vi "Tank Fill.vi"() -> ()   [LabVIEW 2014]
panel:
  out "Tank Level N":i32
  in  "Stop Fill":bool
  in  "Start Fill":bool
  out "Bottom Float Switch":bool
  out "Top Float Switch":bool
  out "Tank level":i32(slide) scale=0.0..300.0
  # "Click          to run"
  # "225"
  # "75"
  # "Tank Fill"
  # "Here, there is a 300 gallon mix tank which mixes red dye.  It drains at a constant rate of 50 gal/sec. There is a pump that can add dye at a rate of 100 gal/sec.\nThere are two float switches, which monitor the level in the tank. When the dye level reaches one of the switches, it is activated, and its value becomes true.\n\nYour job is to add this functionality:\nThe pump is activated by the Start Fill button. When this starts, dye gets pumped into the mix tank until it hits the top float switch. Once this switch is reached, the pump turns off.  \nThe tank level decreases until it the level goes below the bottom float switch. At this point, the pump should start back up and restart the cycle. The tank level should oscillate between the two float switches like this until the stop fill button is pushed, at which point the tank will drain."
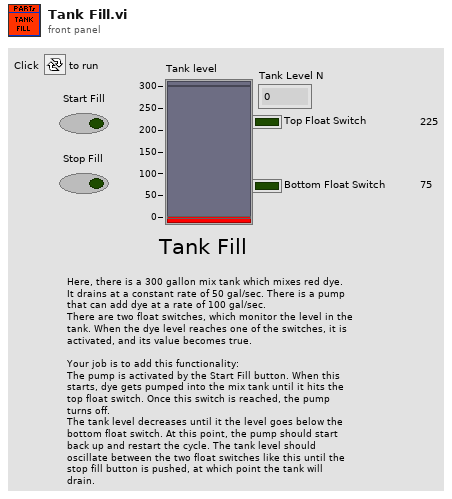
[diagram p1: front panel]
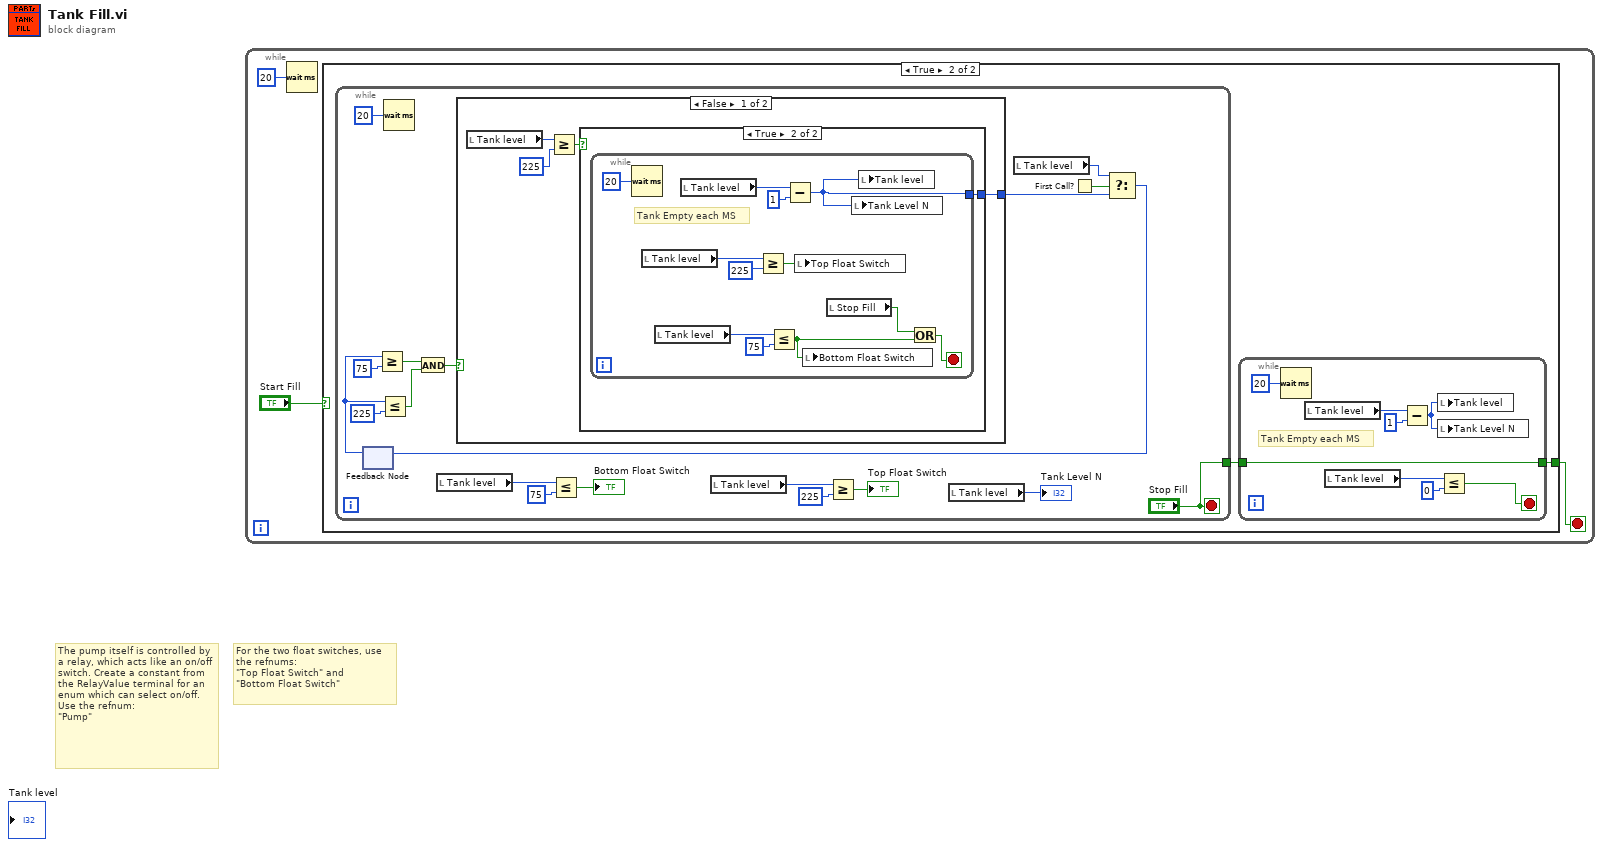
[diagram p0: block diagram]
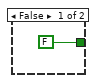
[diagram p2: hidden frame]
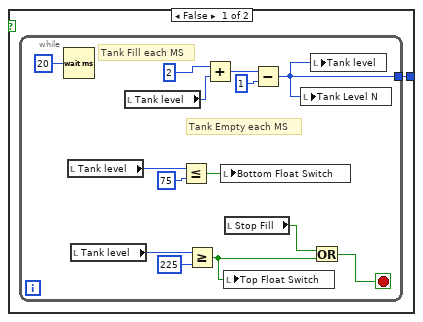
[diagram p3: hidden frame]
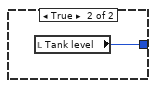
[diagram p4: hidden frame]
diagram:
  # "The pump itself is controlled by a relay, which acts like an on/off switch. Create a constant from the RelayValue terminal for an enum which can select on/off.\nUse the refnum:\n\"Pump\""
  # "For the two float switches, use\nthe refnums:\n\"Top Float Switch\" and\n\"Bottom Float Switch\""
  n1 = while {
    stop <- w2 stop-if-true
    n2 = Wait (ms)(milliseconds to wait=u32 20) -> ()  [unwired: 1 out]
    n3 = case shown="True" "Start Fill" {
      tunnel: [FALSE ("Stop Fill") w5] -> w2
      frame False {
      }
      frame True {
        n4 = while {
          tunnel: ["Stop Fill"] -> w6
          stop <- "Stop Fill" stop-if-true
          n5 = feedback #1() -> (w18:i32)  [unwired: 1 in]
          n6 = Greater Or Equal?(x=w18, y=75) -> (x >= y?=w25:bool)
          n7 = Less Or Equal?(x=w18, y=225) -> (x <= y?=w24:bool)
          n8 = Wait (ms)(milliseconds to wait=u32 20) -> ()  [unwired: 1 out]
          n9 = And(x=w25, y=w24) -> (x .and. y?=w23:bool)
          n10 = local read "Tank level"() -> (w30:i32)
          n11 = case shown="False" w23 {
            tunnel: [w34 w66] -> w20
            frame False {
              n12 = local read "Tank level"() -> (w37:i32)
              n13 = Greater Or Equal?(x=w37, y=225) -> (x >= y?=w35:bool)
              n14 = case shown="True" w35 {
                tunnel: [w38 w53] -> w34
                frame False {
                  n15 = while {
                    tunnel: [w40] -> w38
                    stop <- w41 stop-if-true
                    # "Tank Empty each MS"
                    # "Tank Fill each MS"
                    n16 = Wait (ms)(milliseconds to wait=u32 20) -> ()  [unwired: 1 out]
                    n17 = local read "Tank level"() -> (w45:i32)
                    n18 = local read "Tank level"() -> (w52:i32)
                    n19 = local read "Tank level"() -> (w50:i32)
                    n20 = Less Or Equal?(x=w45, y=75) -> (x <= y?=w44:bool)
                    n21 = Greater Or Equal?(x=w52, y=225) -> (x >= y?=w42:bool)
                    n22 = Add(x=2, y=w50) -> (x+y=w49:i32)
                    n23 = local write "Bottom Float Switch"(w44) -> ()
                    n24 = local write "Top Float Switch"(w42) -> ()
                    n25 = local read "Stop Fill"() -> (w43:bool)
                    n26 = Subtract(x=w49, y=1) -> (x-y=w40:i32)
                    n27 = local write "Tank Level N"(w40) -> ()
                    n28 = local write "Tank level"(w40) -> ()
                    n29 = Or(x=w43, y=w42) -> (x .or. y?=w41:bool)
                  }
                }
                frame True {
                  n30 = while {
                    tunnel: [w58] -> w53
                    stop <- w60 stop-if-true
                    # "Tank Empty each MS"
                    n31 = Wait (ms)(milliseconds to wait=u32 20) -> ()  [unwired: 1 out]
                    n32 = local read "Tank level"() -> (w56:i32)
                    n33 = local read "Tank level"() -> (w65:i32)
                    n34 = local read "Tank level"() -> (w61:i32)
                    n35 = Greater Or Equal?(x=w56, y=225) -> (x >= y?=w54:bool)
                    n36 = Less Or Equal?(x=w65, y=75) -> (x <= y?=w57:bool)
                    n37 = Subtract(x=w61, y=1) -> (x-y=w58:i32)
                    n38 = local write "Top Float Switch"(w54) -> ()
                    n39 = local write "Bottom Float Switch"(w57) -> ()
                    n40 = local read "Stop Fill"() -> (w59:bool)
                    n41 = local write "Tank Level N"(w58) -> ()
                    n42 = local write "Tank level"(w58) -> ()
                    n43 = Or(x=w59, y=w57) -> (x .or. y?=w60:bool)
                  }
                }
              }
            }
            frame True {
              n44 = local read "Tank level"() -> (w66:i32)
            }
          }
          n45 = Less Or Equal?(x=w30, y=75) -> (x <= y?=→"Bottom Float Switch":bool)
          n46 = local read "Tank level"() -> (w32:i32)
          n47 = Greater Or Equal?(x=w32, y=225) -> (x >= y?=→"Top Float Switch":bool)
          n48 = local read "Tank level"() -> (→"Tank Level N":i32)
          n49 = local read "Tank level"() -> (w22:i32)
          n50 = First Call?() -> (First Call?: T/F=w21:bool)
          n51 = Select(t=w22, s=w21, f=w20) -> (s? t:f=w19:i32)
          n52 = feedback-in #1(w19) -> ()
        }
        n53 = while {
          tunnel: w6 -> [w7]
          tunnel: [w7] -> w5
          stop <- w9 stop-if-true
          # "Tank Empty each MS"
          n54 = Wait (ms)(milliseconds to wait=u32 20) -> ()  [unwired: 1 out]
          n55 = local read "Tank level"() -> (w13:i32)
          n56 = local read "Tank level"() -> (w10:i32)
          n57 = Subtract(x=w13, y=1) -> (x-y=w12:i32)
          n58 = local write "Tank level"(w12) -> ()
          n59 = local write "Tank Level N"(w12) -> ()
          n60 = Less Or Equal?(x=w10, y=0) -> (x <= y?=w9:bool)
        }
      }
    }
  }
